vi "PlotFeRfe.vi"(5 "REPlotRef":refnum<vi>, 7 "FEPlotRef":refnum<vi>, 8 "ErrorArray":errorcluster[](array[cluster]), 10 "clPmuImpairRptArray":T1 {"Synx" format="%#_4g"}, 11 "clEvtReportArray":T1 {"Synx" format="%#_4g"}) -> (0 "ErrorArray":errorcluster[](array[cluster]))   [LabVIEW 2014, in "Visualization.lvlib" / "VisualizePMU_class.lvclass"]
uses:
  VisualizePMU_class.lvclass
  Modules/EventPlugins/EventPluginBaseClass/TypeDefs/clEvtReportArray.ctl
  Modules/EventPlugins/EventPluginBaseClass/TypeDefs/clEvtReport.ctl
  Modules/EventPlugins/EventPluginBaseClass/EventPluginBaseClass.lvclass
panel:
  out "RFE Plot":cluster{dbl[], dbl[]}(graph)
  out "FE Plot":cluster{dbl[], dbl[]}(graph)
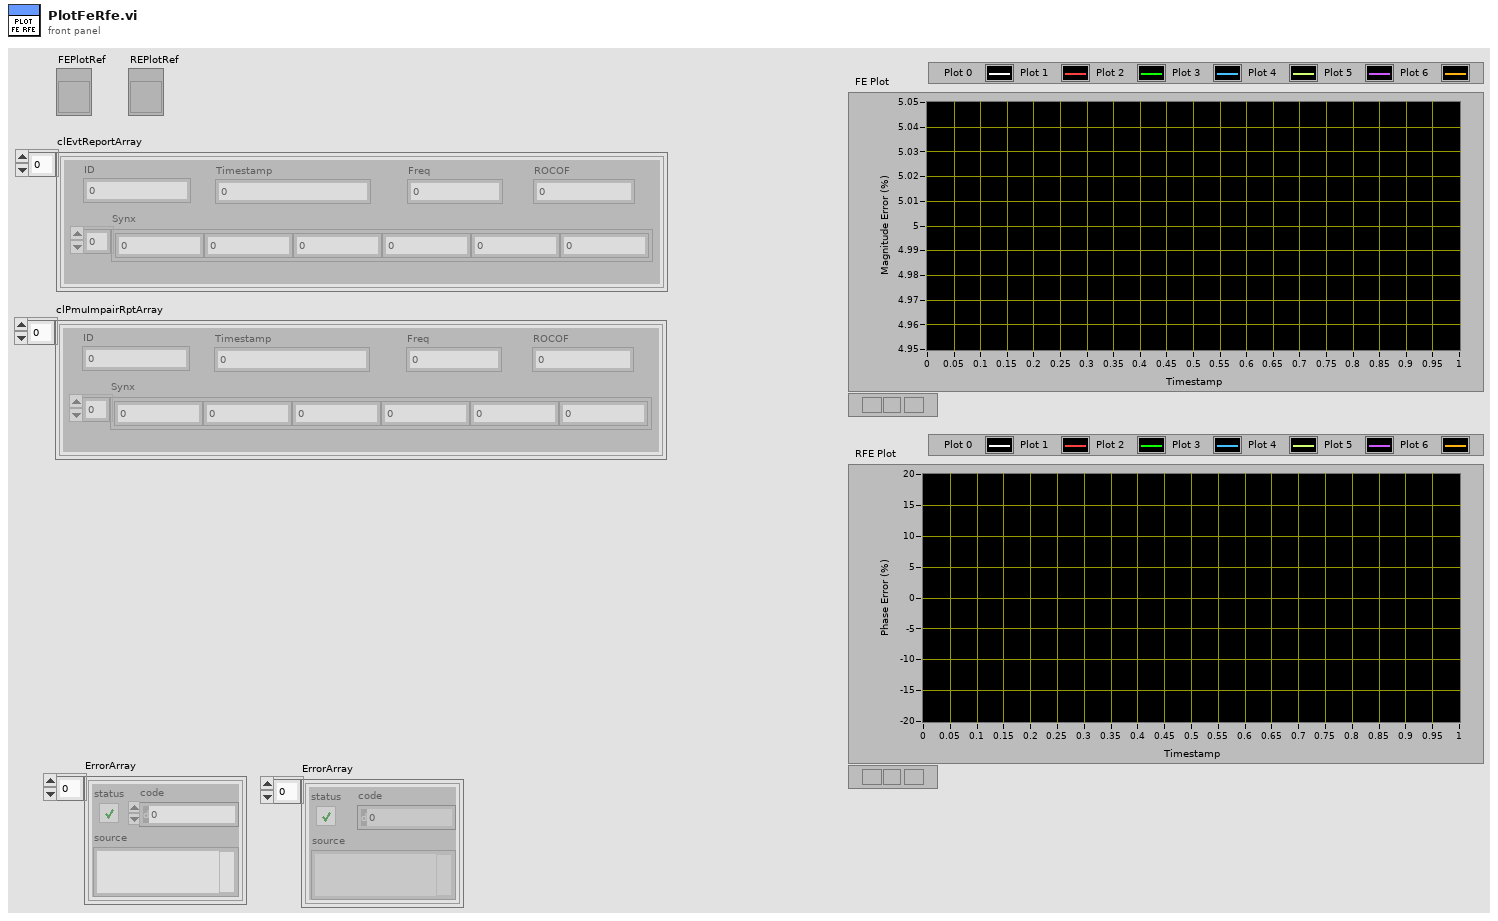
[diagram p1: front panel]
types:
  T1 = typedef "EventPlugins.lvlib/EventPluginBaseClass.lvclass/clEvtReportArray.ctl" = T2[]
  T2 = typedef "EventPlugins.lvlib/EventPluginBaseClass.lvclass/clEvtReport.ctl" = cluster{"Timestamp":dbl, "Synx":cdb[], "Freq":dbl, "ROCOF":dbl, "ID":i16}
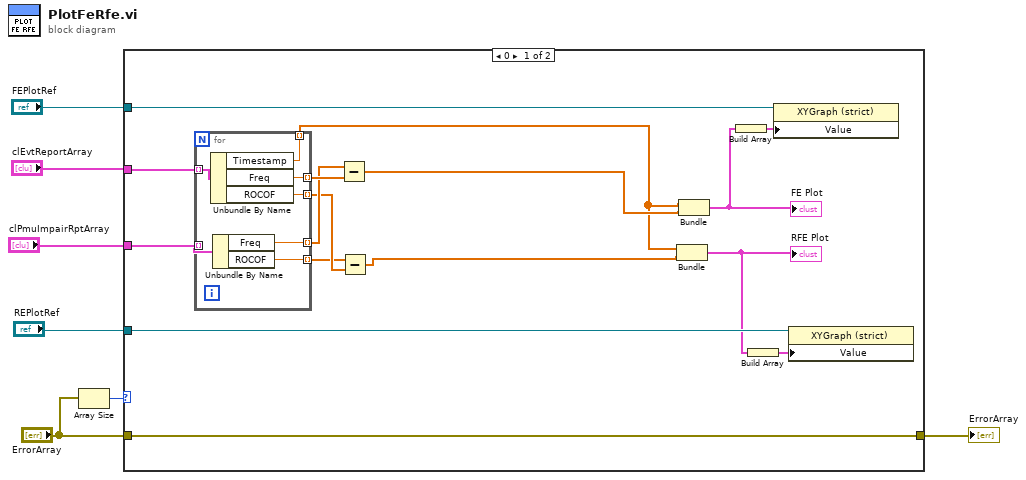
[diagram p0: block diagram]
diagram:
  n1 = Array Size(array="ErrorArray") -> (size(s)=w7:i32)
  n2 = case shown="0" w7 {
    tunnel: "ErrorArray" -> [w15 w31]
    tunnel: [w15 w31] -> w5
    tunnel: "clEvtReportArray" -> [w23 _]
    tunnel: "clPmuImpairRptArray" -> [w22 _]
    tunnel: "FEPlotRef" -> [w21 _]
    tunnel: "REPlotRef" -> [w20 _]
    frame 0 {
      n3 = for {
        tunnel: w22 -> [w30] mode=indexing
        tunnel: w23 -> [w29] mode=indexing
        tunnel: [w28] -> w19 mode=indexing
        tunnel: [w27] -> w18 mode=indexing
        tunnel: [w26] -> w12 mode=indexing
        tunnel: [w25] -> w17 mode=indexing
        tunnel: [w24] -> w16 mode=indexing
        n4 = Unbundle By Name(w29) -> ("Timestamp"=w26:dbl, "Freq"=w28:dbl, "ROCOF"=w25:dbl)
        n5 = Unbundle By Name(w30) -> ("Freq"=w27:dbl, "ROCOF"=w24:dbl)
      }
      n6 = Subtract(x=w18, y=w19) -> (x-y=w14:dbl[])
      n7 = Subtract(x=w16, y=w17) -> (x-y=w13:dbl[])
      n8 = Bundle(w12, w13) -> (w8:cluster{dbl[], dbl[]})  [unwired: 1 in]
      "RFE Plot" <- w8
      n9 = Bundle(w12, w14) -> (w11:cluster{dbl[], dbl[]})  [unwired: 1 in]
      "FE Plot" <- w11
      n10 = Build Array(w11) -> (w10:cluster{dbl[], dbl[]}[])
      n11 = Build Array(w8) -> (w9:cluster{dbl[], dbl[]}[])
      n12 = property class="XYGraph (strict)"(reference=w21, "Value"=w10) -> ()  [unwired: 1 in, 2 out]
      n13 = property class="XYGraph (strict)"(reference=w20, "Value"=w9) -> ()  [unwired: 1 in, 2 out]
    }
    frame 1, Default {
    }
  }
  "ErrorArray" <- w5
